vi "Run Tests.vi"   [LabVIEW 2018]
uses:
  <vilib>/addons/_JKI Toolkits/Caraya/classes/Properties.Assert/Properties.Assert.lvclass
  C:/Program Files (x86)/National Instruments/LabVIEW 2018/vi.lib/addons/_JKI Toolkits/Caraya/classes/Properties/Properties.lvclass
  <vilib>/addons/_JKI Toolkits/Caraya/classes/Assert/Assert Not Error.vi
  <vilib>/addons/_JKI Toolkits/Caraya/classes/Test/Test.lvclass
  TwinCAT ADS Class/TwinCAT ADS.lvclass
  <vilib>/addons/_JKI Toolkits/Caraya/classes/Assert/Assert.lvclass
  <vilib>/addons/_JKI Toolkits/Caraya/classes/Properties/Properties.lvclass
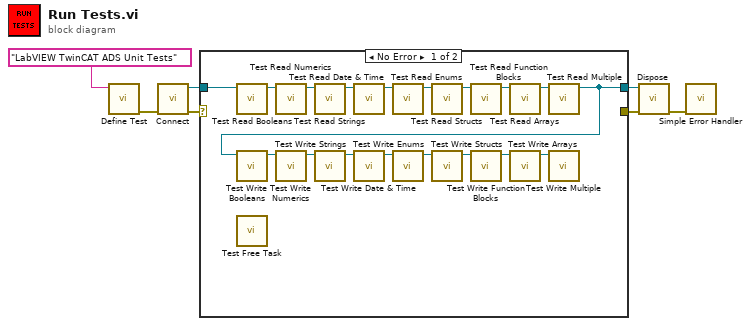
[diagram p0: block diagram]
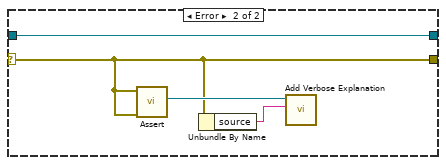
[diagram p2: hidden frame]
diagram:
  n1 = call <vilib>:"Define Test.vi"("Label (VI Title)"="LabVIEW TwinCAT ADS Unit Tests") -> ("error out"=w6:errorcluster)  [unwired: 9 in, 1 out]
  n2 = call "Connect.vi"("error in (no error)"=w6) -> ("error out"=w3:errorcluster, "TwinCAT ADS out"=w7:refnum<class "TwinCAT ADS.lvclass">)  [unwired: 9 in]
  n3 = case shown="No Error" w3 {
    selector: w3 -> [_ w26]
    tunnel: w7 -> [w25 w29]
    tunnel: [w11 w29] -> w5
    tunnel: [_ w26] -> w2
    frame No Error {
      n4 = call "Test Read Booleans.vi"("TwinCAT ADS in"=w25) -> ("TwinCAT ADS out"=w24:refnum<class "TwinCAT ADS.lvclass">)  [unwired: 10 in]
      n5 = call "Test Free Task.vi"() -> ()  [unwired: 12 in]
      n6 = call "Test Read Numerics.vi"("TwinCAT ADS in"=w24) -> ("TwinCAT ADS out"=w23:refnum<class "TwinCAT ADS.lvclass">)  [unwired: 10 in]
      n7 = call "Test Read Strings.vi"("TwinCAT ADS in"=w23) -> ("TwinCAT ADS out"=w22:refnum<class "TwinCAT ADS.lvclass">)  [unwired: 10 in]
      n8 = call "Test Read Date & Time.vi"("TwinCAT ADS in"=w22) -> ("TwinCAT ADS out"=w21:refnum<class "TwinCAT ADS.lvclass">)  [unwired: 10 in]
      n9 = call "Test Read Enums.vi"("TwinCAT ADS in"=w21) -> ("TwinCAT ADS out"=w20:refnum<class "TwinCAT ADS.lvclass">)  [unwired: 10 in]
      n10 = call "Test Read Structs.vi"("TwinCAT ADS in"=w20) -> ("TwinCAT ADS out"=w14:refnum<class "TwinCAT ADS.lvclass">)  [unwired: 10 in]
      n11 = call "Test Read Function Blocks.vi"("TwinCAT ADS in"=w14) -> ("TwinCAT ADS out"=w13:refnum<class "TwinCAT ADS.lvclass">)  [unwired: 10 in]
      n12 = call "Test Read Arrays.vi"("TwinCAT ADS in"=w13) -> ("TwinCAT ADS out"=w12:refnum<class "TwinCAT ADS.lvclass">)  [unwired: 10 in]
      n13 = call "Test Read Multiple.vi"("TwinCAT ADS in"=w12) -> ("TwinCAT ADS out"=w11:refnum<class "TwinCAT ADS.lvclass">)  [unwired: 10 in]
      n14 = call "Test Write Booleans.vi"("TwinCAT ADS in"=w11) -> ("TwinCAT ADS out"=w19:refnum<class "TwinCAT ADS.lvclass">)  [unwired: 10 in]
      n15 = call "Test Write Numerics.vi"("TwinCAT ADS in"=w19) -> ("TwinCAT ADS out"=w18:refnum<class "TwinCAT ADS.lvclass">)  [unwired: 10 in]
      n16 = call "Test Write Strings.vi"("TwinCAT ADS in"=w18) -> ("TwinCAT ADS out"=w16:refnum<class "TwinCAT ADS.lvclass">)  [unwired: 10 in]
      n17 = call "Test Write Date & Time.vi"("TwinCAT ADS in"=w16) -> ("TwinCAT ADS out"=w15:refnum<class "TwinCAT ADS.lvclass">)  [unwired: 10 in]
      n18 = call "Test Write Enums.vi"("TwinCAT ADS in"=w15) -> ("TwinCAT ADS out"=w17:refnum<class "TwinCAT ADS.lvclass">)  [unwired: 10 in]
      n19 = call "Test Write Structs.vi"("TwinCAT ADS in"=w17) -> ("TwinCAT ADS out"=w10:refnum<class "TwinCAT ADS.lvclass">)  [unwired: 10 in]
      n20 = call "Test Write Function Blocks.vi"("TwinCAT ADS in"=w10) -> ("TwinCAT ADS out"=w9:refnum<class "TwinCAT ADS.lvclass">)  [unwired: 10 in]
      n21 = call "Test Write Arrays.vi"("TwinCAT ADS in"=w9) -> ("TwinCAT ADS out"=w8:refnum<class "TwinCAT ADS.lvclass">)  [unwired: 10 in]
      n22 = call "Test Write Multiple.vi"("TwinCAT ADS in"=w8) -> ()  [unwired: 10 in, 1 out]
    }
    frame Error {
      n23 = call-poly <vilib>:"Assert.vi"("error in (no error)"=w26, "Not Error?"=w26) -> ("Properties.Assert"=w28:refnum<class "Properties.Assert.lvclass">)  [unwired: 8 in, 1 out]
      n24 = Unbundle By Name(w26) -> ("source"=w27:string)
      n25 = call <vilib>:"Add Verbose Explanation.vi"("Verbose Explanation"=w27, "Properties"=w28) -> ()  [unwired: 8 in, 2 out]
    }
  }
  n26 = call "Dispose.vi"("error in (no error)"=w2, "TwinCAT ADS in"=w5) -> ("error out"=w1:errorcluster)  [unwired: 9 in]
  n27 = call <vilib>:"Simple Error Handler.vi"("error in (no error)"=w1) -> ()  [unwired: 4 in, 5 out]
